vi "Ini_file_read from file.vi"(0 "config file path":path=path "C:/Labview Projects/Skywire/TestStation.ini", 1 "Operation":T1(ring), 5 "Section Name":string="general", 7 "Key Name":string="test_pc_name", 9 "New key data":string, 11 "error in (no error)":errorcluster) -> (4 "config file path out":path, 6 "Key data from file":string, 8 "KeyFound?":bool, 15 "error out":errorcluster)   [LabVIEW 2013]
uses:
  <vilib>/Utility/config.llb/Write Key (String).vi
  <vilib>/Utility/config.llb/NI_LVConfig.lvlib
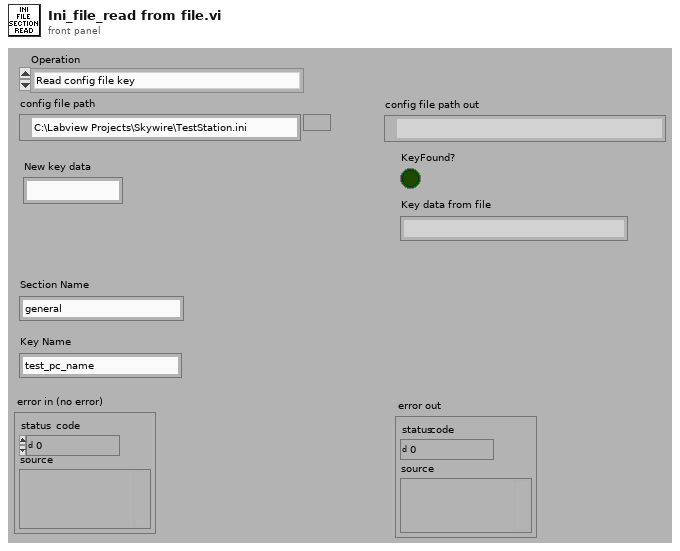
[diagram p1: front panel]
types:
  T1 = enum16{"Read config file key", "Write config file key", "Read config file key and compare"}
  T2 = typedef "NI_LVConfig.lvlib/Config Data RefNum.ctl" = refnum<k1>
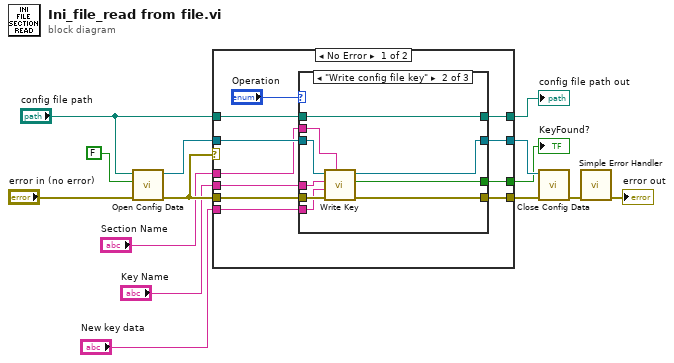
[diagram p0: block diagram]
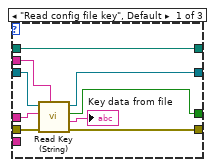
[diagram p2: hidden frame]
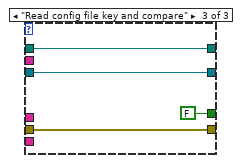
[diagram p3: hidden frame]
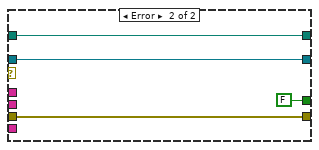
[diagram p4: hidden frame]
diagram:
  n1 = call <vilib>:"Open Config Data.vi"("error in (no error)"="error in (no error)", "create file if necessary (T)"=FALSE, "configuration file path"="config file path") -> ("error out"=w12:errorcluster, "refnum"=w13:T2)  [unwired: 6 in, 1 out]
  n2 = case shown="No Error" w12 {
    tunnel: w13 -> [w24 w50]
    tunnel: [w23 w51] -> w7
    tunnel: w12 -> [w22 w51]
    tunnel: "Section Name" -> [w21 _]
    tunnel: "Key Name" -> [w20 _]
    tunnel: [w19 w50] -> w9
    tunnel: [w18 w49] -> w6
    tunnel: "config file path" -> [w17 w49]
    tunnel: [w16 FALSE ("found?")] -> w2
    tunnel: "New key data" -> [w15 _]
    frame No Error {
      n3 = case shown="\"Write config file key\"" "Operation" {
        tunnel: w24 -> [w34 w41 w44]
        tunnel: [w33 w42 w46] -> w23
        tunnel: w22 -> [w32 w43 w46]
        tunnel: w21 -> [w31 w39 _]
        tunnel: w20 -> [w30 w40 _]
        tunnel: [w29 w38 w44] -> w19
        tunnel: [w28 w35 w47] -> w18
        tunnel: w17 -> [w28 w35 w47]
        tunnel: [w26 w36 FALSE ("found?")] -> w16
        tunnel: w15 -> [_ w37 _]
        frame "Read config file key", Default {
          n4 = call <vilib>:"Read Key (String).vi"("section"=w31, "error in (no error)"=w32, "key"=w30, "refnum"=w34) -> ("error out"=w33:errorcluster, "value"=→"Key data from file":string, "found?"=w26:bool, "refnum out"=w29:T2)  [unwired: 4 in]
        }
        frame "Write config file key" {
          n5 = call-poly <vilib>:"Write Key.vi"("section"=w39, "error in (no error)"=w43, "value"=w37, "key"=w40, "refnum"=w41) -> ("error out"=w42:errorcluster, "found?"=w36:bool, "refnum out"=w38:T2)  [unwired: 4 in]
        }
        frame "Read config file key and compare" {
        }
      }
    }
    frame Error {
    }
  }
  "config file path out" <- w6
  "KeyFound?" <- w2
  n6 = call <vilib>:"Close Config Data.vi"("error in (no error)"=w7, "refnum"=w9) -> ("error out"=w8:errorcluster)  [unwired: 8 in, 1 out]
  n7 = call <vilib>:"Simple Error Handler.vi"("error in (no error)"=w8) -> ("error out"=→"error out":errorcluster)  [unwired: 4 in, 4 out]
